vi "Transform3d_Equals.vi"(9 "otherTransform3d":T1={"TRANSLATION3D"={"X"=0.0, "Y"=0.0, "Z"=0.0}, "ROTATION3D"={"Q_quaternion"={"R"=1.0, "V"=[0.0, 0.0, 0.0]}}} {"TRANSLATION3D"."Z" format="%14.3f"; "TRANSLATION3D"."Y" format="%14.3f"; "TRANSLATION3D"."X" format="%14.3f"}, 11 "inTransform3d":T1={"TRANSLATION3D"={"X"=0.0, "Y"=0.0, "Z"=0.0}, "ROTATION3D"={"Q_quaternion"={"R"=1.0, "V"=[0.0, 0.0, 0.0]}}} {"TRANSLATION3D"."Z" format="%14.3f"; "TRANSLATION3D"."Y" format="%14.3f"; "TRANSLATION3D"."X" format="%14.3f"}) -> (3 "Equals":bool)   [LabVIEW 2019, in "Trajectory_Library.lvlib"]
doc: "Checks equality between this Transform2d and another object.\n\nParameters:\n - IN TRANSFORM - This TRANSFORM data structure\n - OTHER TRANSFORM - The other TRANSFORM to compare \n\nResults:\n - EQUALS - Returns TRUE when both TRANSFORMs are the same."
uses:
  Trajectory_Library.lvlib
  TRANSFORM3D.ctl
  TRANSLATION3D.ctl
  ROTATION3D.ctl
  QUATERNION.ctl
  Rotation3d_GetQuaterion.vi
  Quaternion_Equals.vi
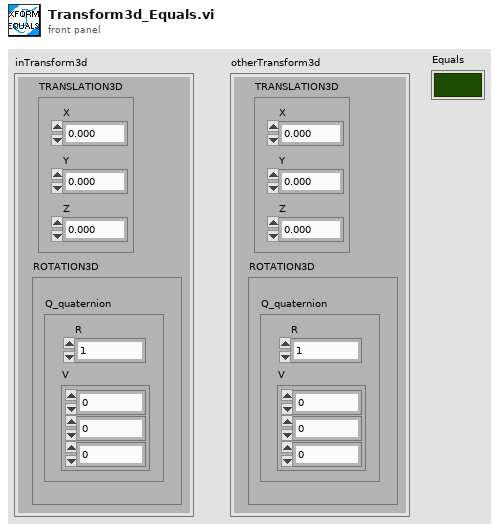
[diagram p1: front panel]
types:
  T1 = typedef "Trajectory_Library.lvlib/TRANSFORM3D.ctl" = cluster{"TRANSLATION3D":T2, "ROTATION3D":T3}
  T2 = typedef "Trajectory_Library.lvlib/TRANSLATION3D.ctl" = cluster{"X":dbl, "Y":dbl, "Z":dbl}
  T3 = typedef "Trajectory_Library.lvlib/ROTATION3D.ctl" = cluster{"Q_quaternion":T4}
  T4 = typedef "Trajectory_Library.lvlib/QUATERNION.ctl" = cluster{"R":dbl, "V":dbl[]}
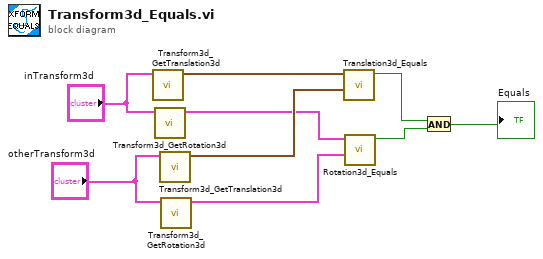
[diagram p0: block diagram]
diagram:
  n1 = call "Transform3d_GetTranslation3d.vi"("in Transform3d"="inTransform3d") -> ("Translation3d"=w4:T2)  [unwired: 10 in]
  n2 = call "Transform3d_GetRotation3d.vi"("in Transform3d"="inTransform3d") -> ("Rotation3d"=w2:T3)  [unwired: 10 in]
  n3 = call "Transform3d_GetTranslation3d.vi"("in Transform3d"="otherTransform3d") -> ("Translation3d"=w3:T2)  [unwired: 10 in]
  n4 = call "Transform3d_GetRotation3d.vi"("in Transform3d"="otherTransform3d") -> ("Rotation3d"=w1:T3)  [unwired: 10 in]
  n5 = call "Translation3d_Equals.vi"("other Translation3d"=w3, "In Translation3d"=w4) -> ("Equals"=w9:bool)  [unwired: 9 in]
  n6 = call "Rotation3d_Equals.vi"("other Rotation3d"=w1, "in Rotation3d"=w2) -> ("Equals"=w8:bool)  [unwired: 9 in]
  n7 = And(x=w9, y=w8) -> (x .and. y?=→"Equals":bool)
